vi "WPI_RobotDriveMotors.vi"(8 "error in (no error)":errorcluster, 9 "RightSpeed":dbl, 10 "LeftSpeed":dbl, 11 "RobotDriveDevRef":T1={"DevStatus"={"status"=FALSE, "code"=0, "source"=""}, "Motors[]"=[], "Square Inputs"=FALSE, "Max Output"=1.0}) -> (0 "error out":errorcluster, 2 "Motor Values":dbl[](array[numeric]), 3 "RobotDriveDevRef":T1={"DevStatus"={"status"=FALSE, "code"=0, "source"=""}, "Motors[]"=[], "Square Inputs"=FALSE, "Max Output"=1.0})   [LabVIEW 2017]
doc: "Determines the motor configuration and sends the speed values to the appropriate left and right motors. Works for 2, 4, 6, and 8 motors provided they are in even/odd slots.\n\nThis software is licensed. Open the labview\\readme\\WPI Robotics Library Open Source License.txt file for more information."
uses:
  <vilib>/Rock Robotics/WPI/RobotDrive/WPI_RobotDriveDevRef.ctl
  <vilib>/Rock Robotics/WPI/MotorControl/WPI_MotorControlDeviceRef.ctl
  <vilib>/Rock Robotics/WPI/MotorControl/WPI_MotorControlType.ctl
  <vilib>/Rock Robotics/SystemInterfaces/DIO/FPGA_DIOPWMChannel.ctl
  <vilib>/Rock Robotics/WPI/PWM/WPI_PWMDeadband.ctl
  <vilib>/Rock Robotics/SystemInterfaces/DIO/FPGA_DIOChannel.ctl
  <vilib>/Rock Robotics/WPI/RobotDrive/WPI_RobotDriveSafetyCheck.vi
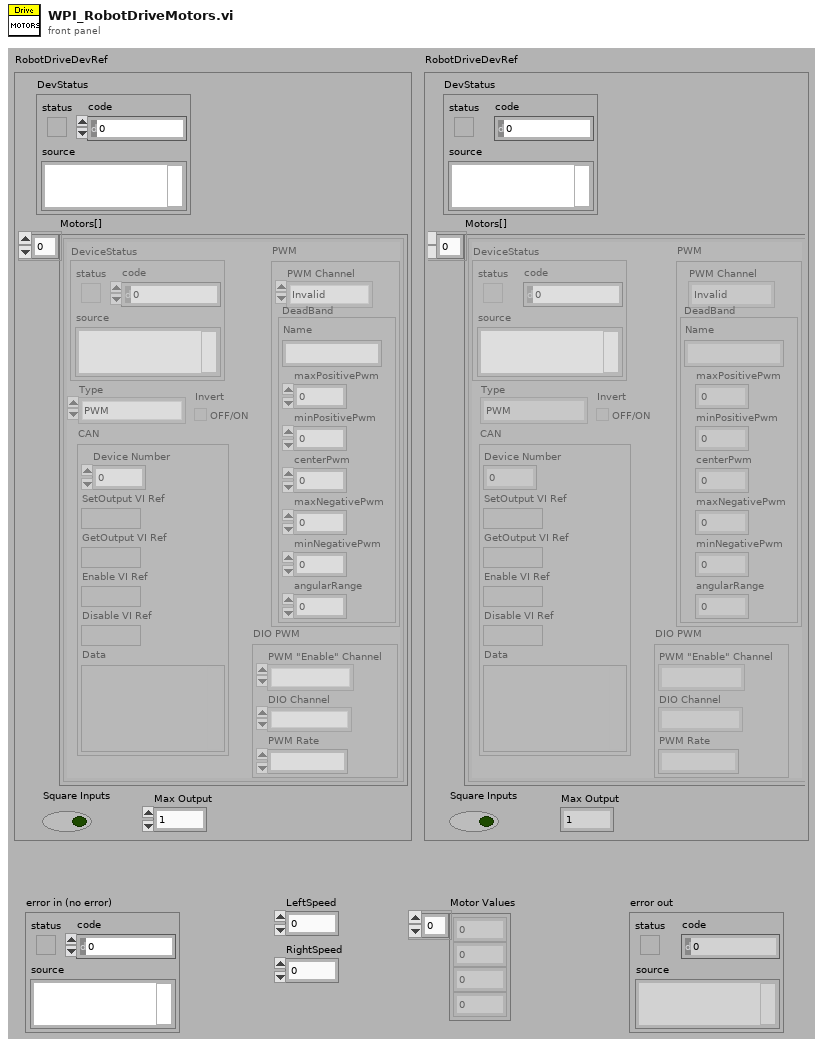
[diagram p1: front panel]
types:
  T1 = typedef "WPI_RobotDriveDevRef.ctl" = cluster{"DevStatus":errorcluster, "Motors[]":T2[], "Square Inputs":bool, "Max Output":dbl}
  T2 = typedef "WPI_MotorControlDeviceRef.ctl" = cluster{"DeviceStatus":errorcluster, "Type":T3, "PWM":cluster{"PWM Channel":T4, "DeadBand":T5}, "CAN":cluster{"Device Number":u8, "SetOutput VI Ref":variant, "GetOutput VI Ref":variant, "Enable VI Ref":variant, "Disable VI Ref":variant, "Data":variant}, "Invert":bool, "DIO PWM":cluster{"PWM \"Enable\" Channel":T4, "DIOChannel":T6, "PWM Rate":dbl}}
  T3 = typedef "WPI_MotorControlType.ctl" = enum16{"PWM", "CAN", "DIO PWM"}
  T4 = typedef "FPGA_DIOPWMChannel.ctl" = enum8{"PWM 0", "PWM 1", "PWM 2", "PWM 3", "PWM 4", "PWM 5", "PWM 6", "PWM 7", "PWM 8", "PWM 9", "PWM MXP 0", "PWM MXP 1", "PWM MXP 2", "PWM MXP 3", "PWM MXP 4", "PWM MXP 5", "PWM MXP 6", "PWM MXP 7", "PWM MXP 8", "PWM MXP 9", "Invalid"}
  T5 = typedef "WPI_PWMDeadband.ctl" = cluster{"Name":string, "maxPositivePwm":i32, "minPositivePwm":i32, "centerPwm":i32, "maxNegativePwm":i32, "minNegativePwm":i32, "angularRange":u16}
  T6 = typedef "FPGA_DIOChannel.ctl" = enum8{"DIO 0", "DIO 1", "DIO 2", "DIO 3", "DIO 4", "DIO 5", "DIO 6", "DIO 7", "DIO 8", "DIO 9", "DIO MXP 0", "DIO MXP 1", "DIO MXP 2", "DIO MXP 3", "DIO MXP 4", "DIO MXP 5", "DIO MXP 6", "DIO MXP 7", "DIO MXP 8", "DIO MXP 9", "DIO MXP 10", "DIO MXP 11", "DIO MXP 12", "DIO MXP 13", "DIO MXP 14", "DIO MXP 15", "SPI Port CS1", "SPI Port CS2", "SPI Port CS3", "SPI Port MISO", "SPI Port MOSI", "Invalid"}
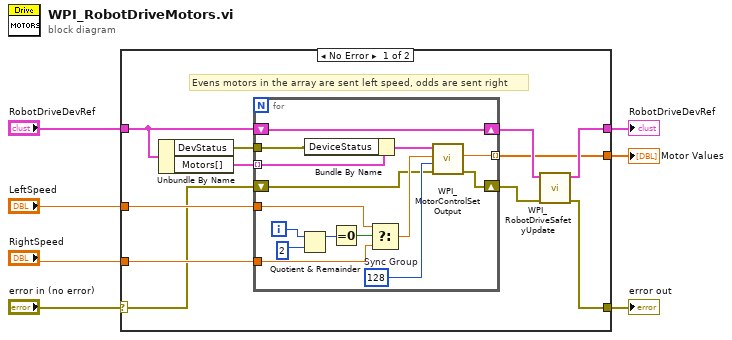
[diagram p0: block diagram]
diagram:
  n1 = case shown="No Error" "error in (no error)" {
    selector: "error in (no error)" -> [w8 w35]
    tunnel: "RobotDriveDevRef" -> [w11 w34]
    tunnel: [w17 w34] -> w6
    tunnel: "LeftSpeed" -> [w16 _]
    tunnel: "RightSpeed" -> [w15 _]
    tunnel: [w18 w35] -> w2
    tunnel: [w12 _] -> w1
    frame No Error {
      # "Evens motors in the array are sent left speed, odds are sent right"
      n2 = Unbundle By Name(w11) -> ("DevStatus"=w9:errorcluster, "Motors[]"=w10:T2[])
      n3 = for {
        tunnel: w16 -> [w29]
        tunnel: w15 -> [w28]
        tunnel: [w25] -> w12 mode=indexing
        shift-right: [w24] -> w14
        shift-left: w8 -> [w23]
        shift-right: [w22] -> w13
        shift-left: w11 -> [w22]
        tunnel: w10 -> [w19] mode=indexing
        tunnel: w9 -> [w20]
        i -> [w32]
        w26 = u8 128  # Sync Group
        n4 = Quotient & Remainder(x=w32, y=2) -> (x-y*floor(x/y)=w31:i32)  [unwired: 1 out]
        n5 = Bundle By Name(cluster=w19, "DeviceStatus"=w20) -> (w21:T2)
        n6 = Equal To 0?(x=w31) -> (x = 0?=w30:bool)
        n7 = Select(t=w29, s=w30, f=w28) -> (s? t:f=w27:dbl)
        n8 = call <vilib>:"WPI_MotorControlSetOutput.vi"("error in (no error)"=w23, "options"=w26, "Output"=w27, "MotorControlDevRef"=w21) -> ("error out"=w24:errorcluster, "Motor Output"=w25:dbl)  [unwired: 1 in, 5 out]
      }
      n9 = call <vilib>:"WPI_RobotDriveSafetyUpdate.vi"("error in (no error)"=w14, "RobotDriveDevRef"=w13) -> ("error out"=w18:errorcluster, "RobotDriveDevRef"=w17:T1)  [unwired: 8 out]
    }
    frame Error {
    }
  }
  "RobotDriveDevRef" <- w6
  "error out" <- w2
  "Motor Values" <- w1
